vi "azura_FitGuassians.vi"(8 "error in":errorcluster caption="entrée d'erreur (pas d'erreur)", 9 "x":dbl[](array[numeric])=array[19206 elements], 10 "Y":dbl[](array[numeric])=array[19206 elements], 11 "Initial param":T1(array[cluster])=[{"Name"="a", "Value"=0.0, "Fit?"=FALSE}, {"Name"="b", "Value"=0.0, "Fit?"=FALSE}, {"Name"="c", "Value"=0.0, "Fit?"=FALSE}, {"Name"="GA1", "Value"=27.0, "Fit?"=TRUE}, {"Name"="GB1", "Value"=3.98, "Fit?"=TRUE}, {"Name"="GC1", "Value"=0.02, "Fit?"=TRUE}, {"Name"="GA2", "Value"=12.0, "Fit?"=TRUE}, {"Name"="GB2", "Value"=4.5, "Fit?"=TRUE}, {"Name"="GC2", "Value"=0.02, "Fit?"=TRUE}, {"Name"="GA3", "Value"=8.0, "Fit?"=TRUE}, {"Name"="GB3", "Value"=8.0, "Fit?"=TRUE}, {"Name"="GC3", "Value"=0.01, "Fit?"=TRUE}] caption="Parameter Name     Guess        Fit?") -> (0 "error out":errorcluster, 1 "Y-fit":cluster{cdb[]}[](graph), 2 "BestFit":cluster{"Name":string, "Parameter":dbl}[](array[cluster])=[{"Name"="GA1", "Parameter"=27.11020289303305}, {"Name"="GB1", "Parameter"=3.9796607658567047}, {"Name"="GC1", "Parameter"=0.03581241758768218}, {"Name"="GA2", "Parameter"=11.731549539598355}, {"Name"="GB2", "Parameter"=4.583557886123198}, {"Name"="GC2", "Parameter"=0.04300288014904538}, {"Name"="GA3", "Parameter"=8.001061678499969}, {"Name"="GB3", "Parameter"=7.5985262902103}, {"Name"="GC3", "Parameter"=-0.06279572775190759}] caption="Parameter Name          best Fit" {"Parameter" format="%.6f"}, 3 "XY Graph":cluster{cdb[]}[](graph), 4 "residue":dbl caption="résidu")   [LabVIEW 2019]
uses:
  <vilib>/gmath/NumericalOptimization/Nonlinear Curve Fit LM.vi
  <vilib>/gmath/NI_Gmath.lvlib
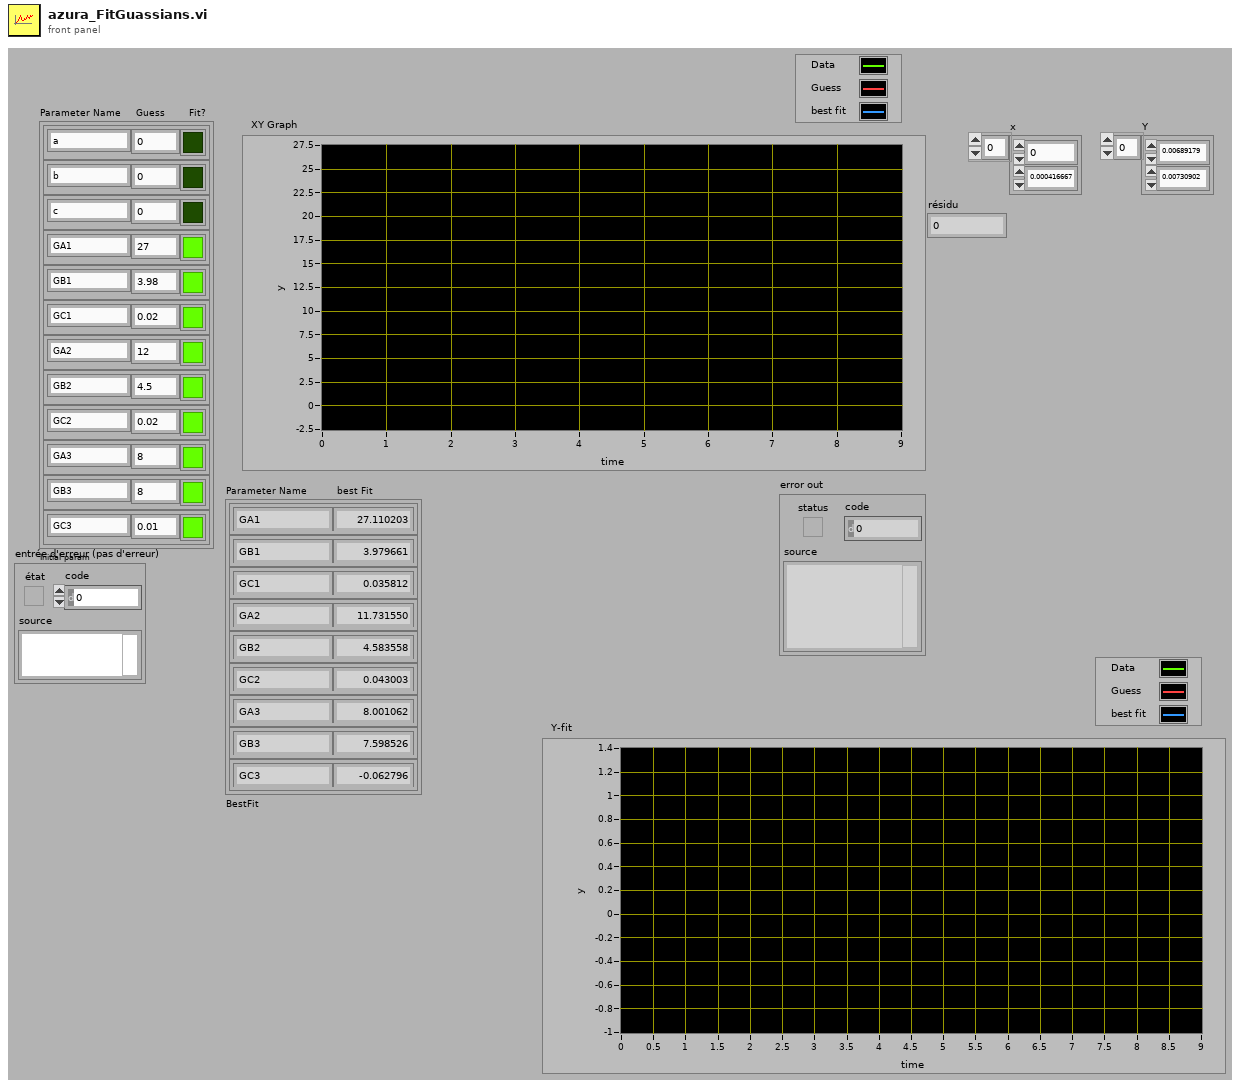
[diagram p1: front panel]
types:
  T1 = cluster{"Name":string, "Value":dbl, "Fit?":bool}[]
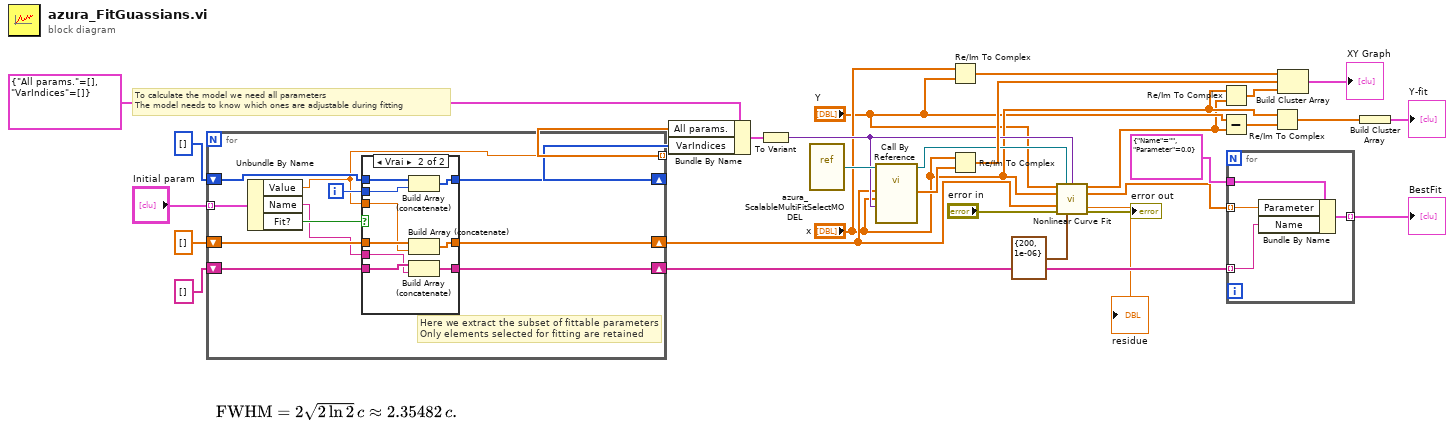
[diagram p0: block diagram]
diagram:
  # "To calculate the model we need all parameters\nThe model needs to know which ones are adjustable during fitting"
  n1 = for {
    shift-right: [w42] -> w14
    shift-left: dbl[] [] -> [w41]
    tunnel: "Initial param" -> [w40] mode=indexing
    tunnel: [w33] -> w22 mode=indexing
    shift-right: [w38] -> w21
    shift-left: i32[] [] -> [w37]
    shift-right: [w34] -> w12
    shift-left: string[] [] -> [w35]
    i -> [w36]
    # "Here we extract the subset of fittable parameters\nOnly elements selected for fitting are retained"
    n2 = Unbundle By Name(w40) -> ("Value"=w33:dbl, "Name"=w32:string, "Fit?"=w39:bool)
    n3 = case shown="Vrai" w39 {
      tunnel: [w45 w53] -> w42
      tunnel: w41 -> [w45 w54]
      tunnel: w33 -> [_ w52]
      tunnel: [w44 w51] -> w38
      tunnel: w37 -> [w44 w50]
      tunnel: w36 -> [_ w49]
      tunnel: [w43 w47] -> w34
      tunnel: w35 -> [w43 w48]
      tunnel: w32 -> [_ w46]
      frame False {
      }
      frame True {
        n4 = Build Array (concatenate)(w50, w49) -> (w51:i32[])
        n5 = Build Array (concatenate)(w54, w52) -> (w53:dbl[])
        n6 = Build Array (concatenate)(w48, w46) -> (w47:string[])
      }
    }
  }
  n7 = Bundle By Name(cluster=cluster{"All params.":dbl[], "VarIndices":i32[]} {"All params."=[], "VarIndices"=[]}, "All params."=w22, "VarIndices"=w21) -> (w24:cluster{"All params.":dbl[], "VarIndices":i32[]})
  n8 = To Variant(anything=w24) -> (Variant=w15:variant)
  n9 = vi-ref "azura_ScalableMultiFitSelectMODEL.vi"() -> (w31:refnum<vi>)
  n10 = call-by-ref "?"(reference=w31, "data"=w15, "x"="x", "a"=w14) -> (reference out=w13:refnum<vi>, "f(X, a)"=w25:dbl[])  [unwired: 2 in, 3 out]
  n11 = Re/Im To Complex(1:"Y", 2:"x") -> (0:w29:cdb[])
  n12 = Re/Im To Complex(1:w25, 2:"x") -> (0:w27:cdb[])
  n13 = call-poly <vilib>:"Nonlinear Curve Fit.vi"("Y"="Y", "f(x,a)"=w13, "data"=w15, "X"="x", "initial parameters"=w14, "error in (no error)"="error in", "termination"=cluster{"max iteration":i32, "tolerance":dbl} {"max iteration"=200, "tolerance"=1e-06}) -> ("best nonlinear fit"=w4:dbl[], "best fit parameters"=w10:dbl[], "residue"=→"residue":dbl, "error out"=→"error out":errorcluster)  [unwired: 3 in, 2 out]
  n14 = Re/Im To Complex(1:w4, 2:"x") -> (0:w26:cdb[])
  n15 = Subtract(x="Y", y=w4) -> (x-y=w3:dbl[])
  n16 = for {
    tunnel: w12 -> [w56] mode=indexing
    tunnel: w10 -> [w58] mode=indexing
    tunnel: cluster{"Name":string, "Parameter":dbl} {"Name"="", "Parameter"=0.0} -> [w57]
    tunnel: [w55] -> w18 mode=indexing
    n17 = Bundle By Name(cluster=w57, "Parameter"=w58, "Name"=w56) -> (w55:cluster{"Name":string, "Parameter":dbl})
  }
  "BestFit" <- w18
  n18 = Re/Im To Complex(1:w3, 2:"x") -> (0:w8:cdb[])
  n19 = Build Cluster Array(w29, w27, w26) -> (→"XY Graph":cluster{cdb[]}[])
  n20 = Build Cluster Array(w8) -> (→"Y-fit":cluster{cdb[]}[])
